vi "Display State 2 Colors.vi"(10 "State In":T2 caption="State") -> (0 "Red BG":T1, 1 "DOF Label":string, 2 "State Out":T2 caption="State", 3 "Units":string, 4 "Red Upper":T1, 5 "Red Lower":T1)   [LabVIEW 2013, in "Limits X.xctl"]
uses:
  Limits X.xctl
  Limits State.ctl
  lib/Data Access Objects/Limits/DofTypes.ctl
  lib/Limits/Limite State.ctl
  lib/Apps/Yes No Button.ctl
  lib/Data Access Objects/Metadata/Persistant DAO Actions.ctl
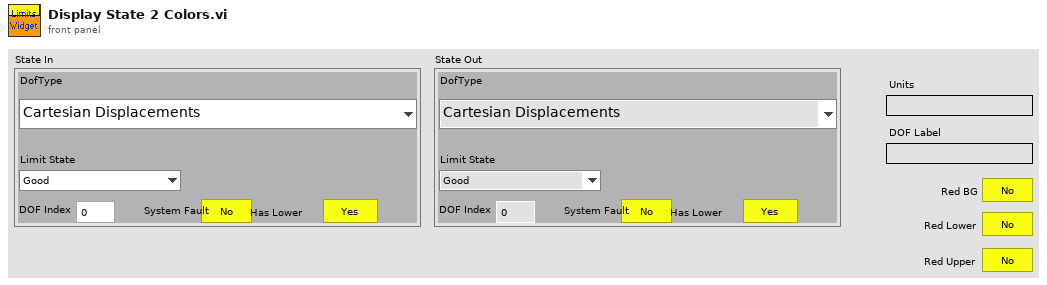
[diagram p1: front panel]
types:
  T1 = typedef "Yes No Button.ctl" = bool
  T2 = typedef "Limits X.xctl/Limits State.ctl" = cluster{"DofType":T3, "Limit State":T4, "DOF Index":i32, "System Fault ":T1, "Has Lower":T1}
  T3 = typedef "DofTypes.ctl" = enum16{"Cartesian Displacements", "Cartesian Forces & Moments", "Actuator Displacements", "Actuator Forces", "Cartesian Increments", "Actuator Increments"}
  T4 = typedef "Limite State.ctl" = enum16{"Good", "Lower Bound Fault", "Upper Bound Fault"}
  T5 = typedef "Persistant DAO Actions.ctl" = enum16{"Init", "Get", "Set", "Load", "Save"}
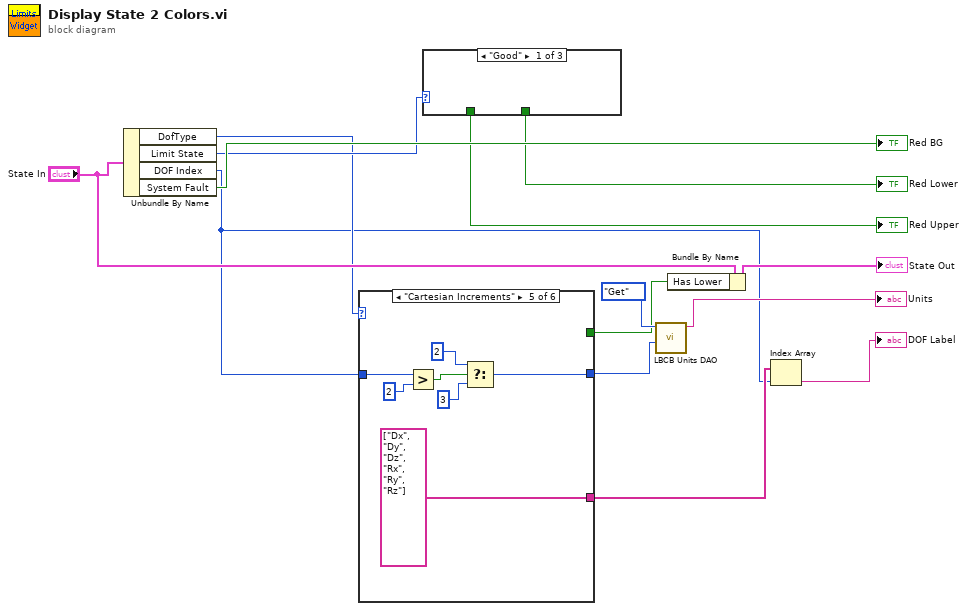
[diagram p0: block diagram]
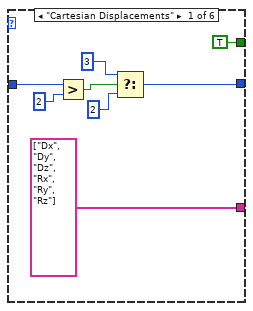
[diagram p2: hidden frame]
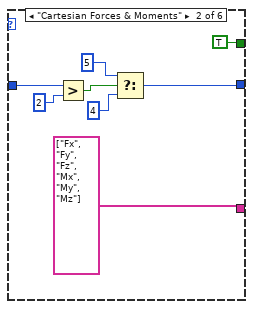
[diagram p3: hidden frame]
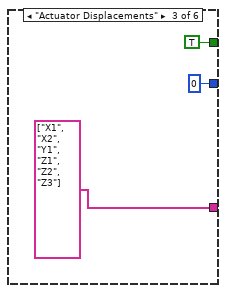
[diagram p4: hidden frame]
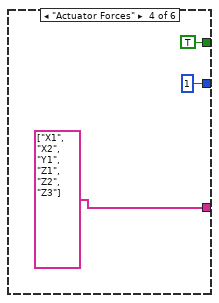
[diagram p5: hidden frame]
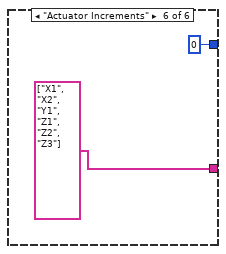
[diagram p6: hidden frame]
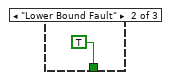
[diagram p7: hidden frame]
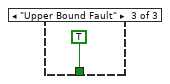
[diagram p8: hidden frame]
diagram:
  n1 = Unbundle By Name("State In") -> ("DofType"=w8:T3, "Limit State"=w11:T4, "DOF Index"=w3:i32, "System Fault"=→"Red BG":T1)
  n2 = case shown="\"Cartesian Increments\"" w8 {
    tunnel: w3 -> [w22 w30 _ _ w43 _]
    tunnel: [w17 w25 0 ("f") 1 ("f") w38 0 ("f")] -> w6
    tunnel: [string[] ["Dx", "Dy", "Dz", "Rx", "Ry", "Rz"] string[] ["Fx", "Fy", "Fz", "Mx", "My", "Mz"] string[] ["X1", "X2", "Y1", "Z1", "Z2", "Z3"] string[] ["X1", "X2", "Y1", "Z1", "Z2", "Z3"] string[] ["Dx", "Dy", "Dz", "Rx", "Ry", "Rz"] string[] ["X1", "X2", "Y1", "Z1", "Z2", "Z3"]] -> w4
    tunnel: [TRUE TRUE TRUE TRUE _ _] -> w1
    frame "Cartesian Displacements" {
      n3 = Greater?(x=w22, y=2) -> (0:w21:bool)
      n4 = Select(t=3, s=w21, f=2) -> (s? t:f=w17:i32)
    }
    frame "Cartesian Forces & Moments" {
      n5 = Greater?(x=w30, y=2) -> (0:w29:bool)
      n6 = Select(t=5, s=w29, f=4) -> (s? t:f=w25:i32)
    }
    frame "Actuator Displacements" {
    }
    frame "Actuator Forces" {
    }
    frame "Cartesian Increments" {
      n7 = Greater?(x=w43, y=2) -> (0:w42:bool)
      n8 = Select(t=2, s=w42, f=3) -> (s? t:f=w38:i32)
    }
    frame "Actuator Increments" {
    }
  }
  n9 = case shown="\"Good\"" w11 {
    tunnel: [_ TRUE _] -> w10
    tunnel: [_ _ TRUE] -> w9
    frame "Good" {
    }
    frame "Lower Bound Fault" {
    }
    frame "Upper Bound Fault" {
    }
  }
  "Red Lower" <- w10
  "Red Upper" <- w9
  n10 = call "LBCB Units DAO.vi"("Index"=w6, "Persistent DAO Actions"=Persistant_DAO_Actions."Get") -> ("Unit"=→"Units":string)  [unwired: 5 in, 4 out]
  n11 = Bundle By Name(cluster="State In", "Has Lower"=w1) -> (→"State Out":T2)
  n12 = Index Array(array=w4, index=w3) -> (element=→"DOF Label":string)
